vi "Async VI Call Template.vi"() -> ()   [LabVIEW 2014]
panel:
  out "error out":errorcluster
  in  "error in (no error)":errorcluster
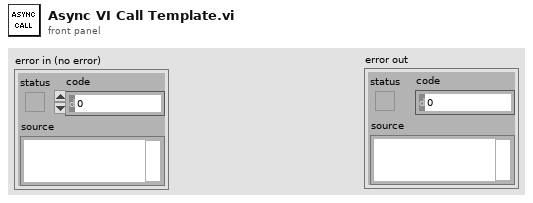
[diagram p1: front panel]
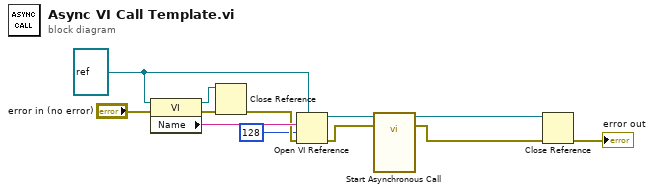
[diagram p0: block diagram]
diagram:
  w1 = refnum<vi> refnum ("type specifier VI Refnum (for type only)")
  n1 = property class="VI"(reference=w1, error in="error in (no error)") -> (reference out=w9:refnum<vi>, error out=w8:errorcluster, "Name"=w11:string)
  n2 = Close Reference(reference=w9, error in (no error)=w8) -> (error out=w7:errorcluster)
  n3 = Open VI Reference(type specifier VI Refnum (for type only)=w1, vi path=w11, options=128, error in (no error)=w7) -> (vi reference=w2:refnum<vi>, error out=w5:errorcluster)  [unwired: 2 in]
  n4 = call-by-ref "Start Asynchronous Call"(reference=w2, error in=w5) -> (reference out=w3:refnum<vi>, error out=w4:errorcluster)
  n5 = Close Reference(reference=w3, error in (no error)=w4) -> (error out=→"error out":errorcluster)
